vi "Hello World.vi"(10 "message":string="Hello World!") -> ()   [LabVIEW 2017]
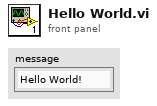
[diagram p1: front panel]
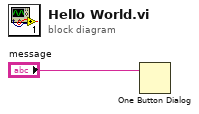
[diagram p0: block diagram]
diagram:
  n1 = One Button Dialog(message="message") -> ()  [unwired: 1 in, 1 out]
